vi "Grid_do_spec.vi"(8 "error in":errorcluster, 9 "FileRefs in":T2, 10 "Settings in":T1={"Drift Correction Settings"={"Drift Correction every"=80, "Drift correction Pixels"=256, "Channel index (0-23)"=0, "MaxImagesBack"=2, "Threshold"=2, "Increment"=8, "max applied Drift Correction"=20, "Correct Drift"=TRUE, "Correlate"=0, "Correct z drift"=FALSE, "zdrift \nDuration (s)"=0.0}, "Spectroscopy Setting"={"Imaging Current"=1e-11, "ref Current"=7e-11, "tip Speed (m/s)"=2e-09, "Imaging Bias"=0.02, "ref Bias"=-0.1, "preSTS delay [ms]"=500, "STS z offset"=2e-10, "during Spec Bias (V)"=-0.1, "trigger1 < Hz"=0.0, "trigger 2 >Hz"=0.0, "autoStop"=FALSE, "Spectroscopy"=0, "PLL ON/OFF"=TRUE, "readjust setpoint every "=1, "z Reference"=FALSE, "Lock In"=TRUE}, "Misc"={"File name"="symmetric_node_zOff=200p", "Email when finished"="cornelius.krull@monash.edu,Dhaneesh.Gopalakrishnan@monash.edu,marina.castelli@monash.edu"}, "Grid Settings"={"type"=1, "type order"=1, "X pixel"=0, "Y pixel"=0, "Grid_Parms"={"center X (m)"=0.0, "center Y (m)"=0.0, "width (m)"=0.0, "height (m)"=0.0, "angle (deg)"=0.0}}} {"Grid Settings"."type order" items=["Line", "Grid"]; "Grid Settings"."type" items=["Line", "Grid"]; "Spectroscopy Setting"."Spectroscopy" items=["Bias", "zSpec"]; "Spectroscopy Setting"."trigger 2 >Hz" format="%#_6p"; "Spectroscopy Setting"."trigger1 < Hz" format="%#_6p"; "Spectroscopy Setting"."during Spec Bias (V)" format="%#_5p"; "Spectroscopy Setting"."STS z offset" format="%#_6p"; "Spectroscopy Setting"."ref Bias" format="%#_6p"; "Spectroscopy Setting"."Imaging Bias" format="%#_6p"; "Spectroscopy Setting"."tip Speed (m/s)" format="%.2p"; "Spectroscopy Setting"."ref Current" format="%#_6p"; "Spectroscopy Setting"."Imaging Current" format="%#_6p"; "Drift Correction Settings"."Correlate" items=["first Frame", "successive Frames"]; "Drift Correction Settings"."max applied Drift Correction" min=1 max=100 step=1 format="%.0p"; "Drift Correction Settings"."Threshold" min=1 step=1; "Drift Correction Settings"."Channel index (0-23)" items=["Current"=0, "Z (m)"=14]}, 11 "Application ref in":refnum<vi>) -> (0 "error out":errorcluster, 1 "FileRefs out":T2, 2 "Settings out":T1={"Drift Correction Settings"={"Drift Correction every"=80, "Drift correction Pixels"=256, "Channel index (0-23)"=0, "MaxImagesBack"=2, "Threshold"=2, "Increment"=8, "max applied Drift Correction"=20, "Correct Drift"=TRUE, "Correlate"=0, "Correct z drift"=FALSE, "zdrift \nDuration (s)"=0.0}, "Spectroscopy Setting"={"Imaging Current"=1e-11, "ref Current"=7e-11, "tip Speed (m/s)"=2e-09, "Imaging Bias"=0.02, "ref Bias"=-0.1, "preSTS delay [ms]"=500, "STS z offset"=2e-10, "during Spec Bias (V)"=-0.1, "trigger1 < Hz"=0.0, "trigger 2 >Hz"=0.0, "autoStop"=FALSE, "Spectroscopy"=0, "PLL ON/OFF"=TRUE, "readjust setpoint every "=1, "z Reference"=FALSE, "Lock In"=TRUE}, "Misc"={"File name"="symmetric_node_zOff=200p", "Email when finished"="cornelius.krull@monash.edu,Dhaneesh.Gopalakrishnan@monash.edu,marina.castelli@monash.edu"}, "Grid Settings"={"type"=1, "type order"=1, "X pixel"=0, "Y pixel"=0, "Grid_Parms"={"center X (m)"=0.0, "center Y (m)"=0.0, "width (m)"=0.0, "height (m)"=0.0, "angle (deg)"=0.0}}} {"Grid Settings"."type order" items=["Line", "Grid"]; "Grid Settings"."type" items=["Line", "Grid"]; "Spectroscopy Setting"."Spectroscopy" items=["Bias", "zSpec"]; "Spectroscopy Setting"."trigger 2 >Hz" format="%#_6p"; "Spectroscopy Setting"."trigger1 < Hz" format="%#_6p"; "Spectroscopy Setting"."during Spec Bias (V)" format="%#_5p"; "Spectroscopy Setting"."STS z offset" format="%#_6p"; "Spectroscopy Setting"."ref Bias" format="%#_6p"; "Spectroscopy Setting"."Imaging Bias" format="%#_6p"; "Spectroscopy Setting"."tip Speed (m/s)" format="%.2p"; "Spectroscopy Setting"."ref Current" format="%#_6p"; "Spectroscopy Setting"."Imaging Current" format="%#_6p"; "Drift Correction Settings"."Correlate" items=["first Frame", "successive Frames"]; "Drift Correction Settings"."max applied Drift Correction" min=1 max=100 step=1 format="%.0p"; "Drift Correction Settings"."Threshold" min=1 step=1; "Drift Correction Settings"."Channel index (0-23)" items=["Current"=0, "Z (m)"=14]}, 3 "Application ref out":refnum<vi>)   [LabVIEW 2014]
uses:
  <userlib>/Nanonis Prog Interface V5/Nanonis Prog Interface.lvlib
panel:
  # "z Spectroscopy"
  # "GRID points"
  # "Increase this if no Drift was detected for \na certain number of images"
  # "% of image size"
  # "z Spectroscopy"
  # "GRID points"
  # "Increase this if no Drift was detected for \na certain number of images"
  # "% of image size"
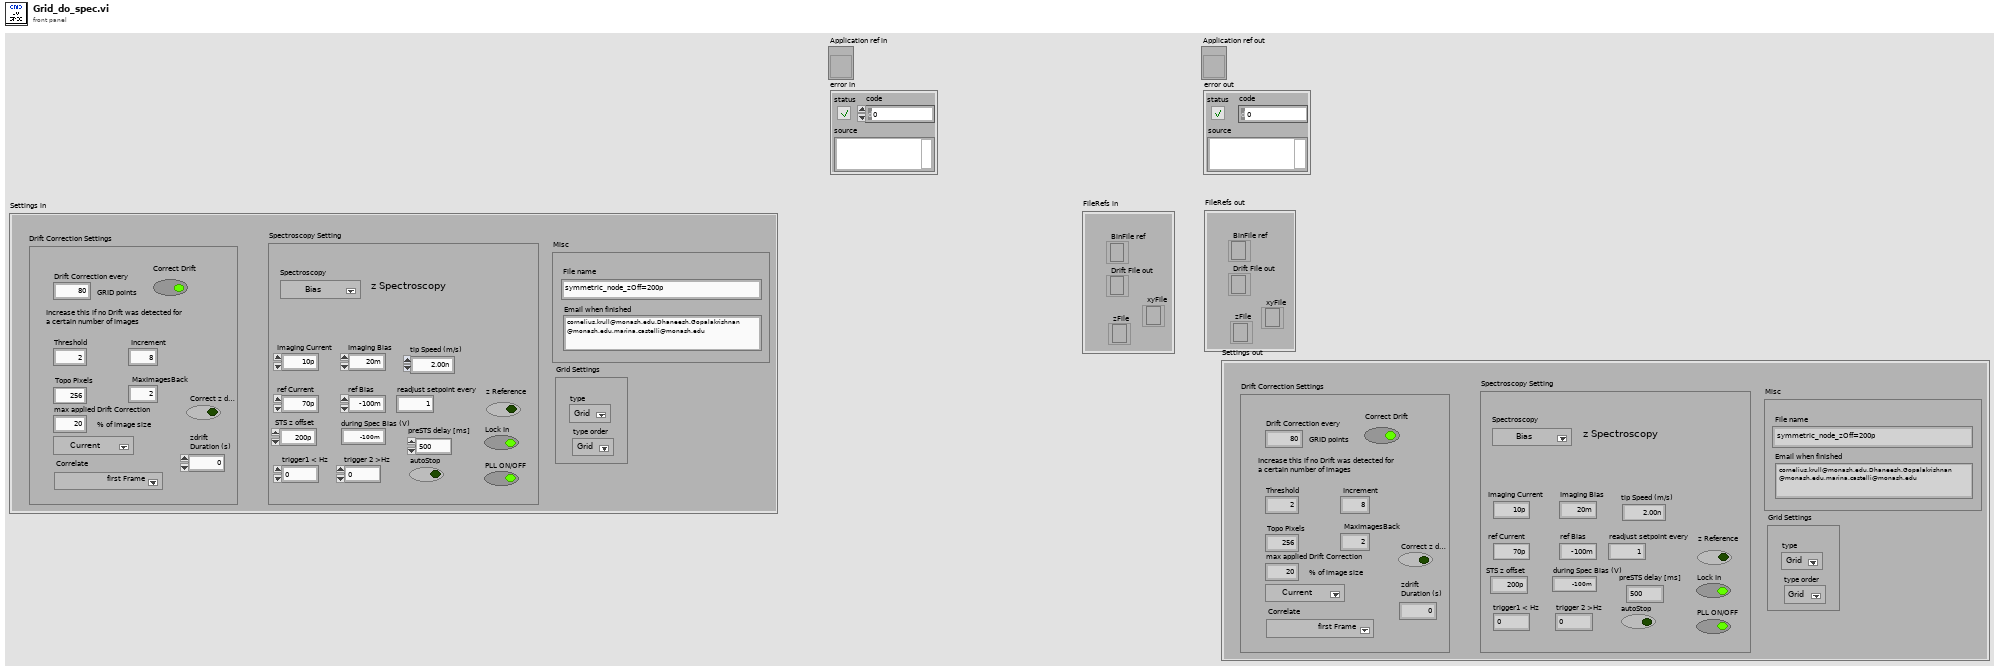
[diagram p1: front panel]
types:
  T1 = cluster{"Drift Correction Settings":cluster{"Drift Correction every":i32, "Drift correction Pixels":i32, "Channel index (0-23)":u8, "MaxImagesBack":i32, "Threshold":i32, "Increment":i32, "max applied Drift Correction":i32, "Correct Drift":bool, "Correlate":u16, "Correct z drift":bool, "zdrift \nDuration (s)":dbl}, "Spectroscopy Setting":cluster{"Imaging Current":dbl, "ref Current":dbl, "tip Speed (m/s)":sgl, "Imaging Bias":dbl, "ref Bias":dbl, "preSTS delay [ms]":u32, "STS z offset":dbl, "during Spec Bias (V)":sgl, "trigger1 < Hz":sgl, "trigger 2 >Hz":sgl, "autoStop":bool, "Spectroscopy":u16, "PLL ON/OFF":bool, "readjust setpoint every ":i32, "z Reference":bool, "Lock In":bool}, "Misc":cluster{"File name":string, "Email when finished":string}, "Grid Settings":cluster{"type":u16, "type order":u16, "X pixel":i32, "Y pixel":i32, "Grid_Parms":cluster{"center X (m)":sgl, "center Y (m)":sgl, "width (m)":sgl, "height (m)":sgl, "angle (deg)":sgl}}}
  T2 = cluster{"Drift File out":refnum<file>, "zFile":refnum<file>, "BinFile ref":refnum<file>, "xyFile":refnum<file>}
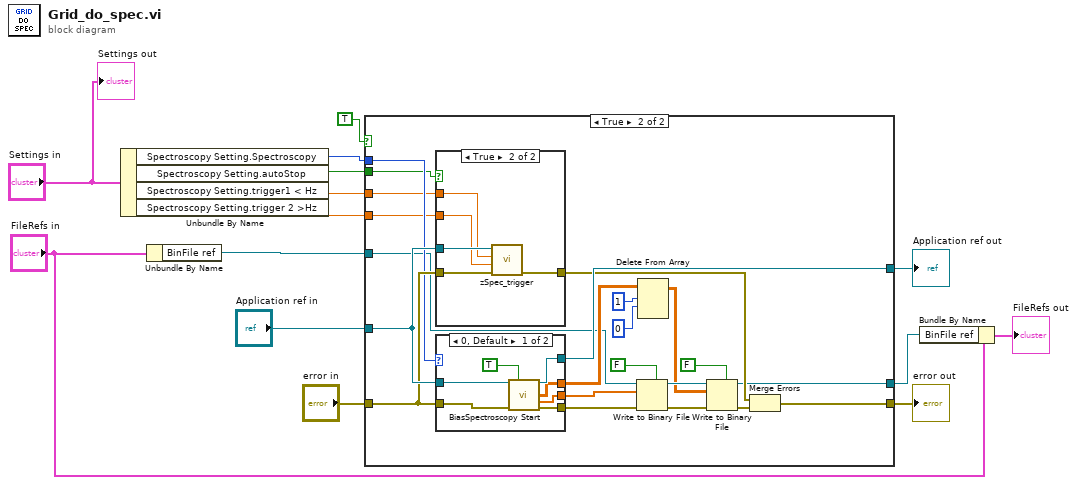
[diagram p0: block diagram]
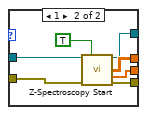
[diagram p3: hidden frame]
diagram:
  n1 = Unbundle By Name("Settings in") -> ("Spectroscopy Setting.Spectroscopy"=w9:u16, "Spectroscopy Setting.autoStop"=w8:bool, "Spectroscopy Setting.trigger1 < Hz"=w2:sgl, "Spectroscopy Setting.trigger 2 >Hz"=w1:sgl)
  n2 = Unbundle By Name("FileRefs in") -> ("BinFile ref"=w7:refnum<file>)
  n3 = case shown="True" TRUE {
    tunnel: [w17 w24] -> w12
    tunnel: "error in" -> [w17 w27]
    tunnel: "Application ref in" -> [w16 w28]
    tunnel: [w16 w29] -> w13
    tunnel: w9 -> [_ w23]
    tunnel: w8 -> [_ w22]
    tunnel: w7 -> [w15 w21]
    tunnel: [w15 w20] -> w4
    tunnel: w2 -> [_ w19]
    tunnel: w1 -> [_ w18]
    frame False {
      # "Point indices aren't multiple of subgrid spacing\n=> no spectroscopy at this point"
    }
    frame True {
      n4 = case shown="True" w22 {
        tunnel: w28 -> [_ w59]
        tunnel: w27 -> [w54 w58]
        tunnel: [w54 w57] -> w26
        tunnel: w19 -> [_ w56]
        tunnel: w18 -> [_ w55]
        frame False {
        }
        frame True {
          n5 = call "zSpec_trigger.vi"("Error in (no error)"=w58, "trigger 2"=w55, "trigger1"=w56, "Application ref in"=w59) -> ("Error out"=w57:errorcluster)  [unwired: 5 in, 1 out]
        }
      }
      n6 = case shown="0, Default" w23 {
        tunnel: [w40 w53] -> w38
        tunnel: [w41 w52] -> w37
        tunnel: [w42 w50] -> w31
        tunnel: [w43 w49] -> w29
        tunnel: w28 -> [w45 w48]
        tunnel: w27 -> [w44 w47]
        frame 0, Default {
          n7 = call <userlib>:"BiasSpectroscopy Start.vi"("Application ref in"=w45, "Get data (F)"=TRUE, "Error in (no error)"=w44) -> ("Application ref out"=w43:refnum<vi>, "Data"=w40:sgl[][], "Parameters"=w41:sgl[], "Error out"=w42:errorcluster)  [unwired: 8 in, 1 out]
        }
        frame 1 {
          n8 = call <userlib>:"Z-Spectroscopy Start.vi"("Application ref in"=w48, "Get data (F=False)"=TRUE ("Get Data (F)"), "error in (no error)"=w47) -> ("Application ref out"=w49:refnum<vi>, "Data"=w53:sgl[][], "Parameters"=w52:sgl[], "error out"=w50:errorcluster)  [unwired: 8 in, 1 out]
        }
      }
      n9 = Write to Binary File(file (use dialog)=w21, data=w37, error in=w31, 5:FALSE ("prepend array or string size? (T)")) -> (refnum out=w39:refnum<file>, error out=w30:errorcluster)  [unwired: 2 in, 1 out]
      n10 = Delete From Array(array=w38, length=1, index (row)=0 ("index")) -> (array with subset deleted=w36:sgl[][])  [unwired: 1 in, 1 out]
      n11 = Write to Binary File(file (use dialog)=w39, data=w36, error in=w30, 5:FALSE ("prepend array or string size? (T)")) -> (refnum out=w20:refnum<file>, error out=w25:errorcluster)  [unwired: 2 in, 1 out]
      n12 = Merge Errors(w26, w25) -> (w24:errorcluster)
    }
  }
  "Application ref out" <- w13
  "error out" <- w12
  n13 = Bundle By Name(cluster="FileRefs in", "BinFile ref"=w4) -> (→"FileRefs out":T2)
  "Settings out" <- "Settings in"
